vi "medicaoIXV.vi"() -> ()   [LabVIEW 2012]
uses:
  <vilib>/Utility/file.llb/Write To Spreadsheet File (string).vi
  <vilib>/Utility/file.llb/Write To Spreadsheet File (DBL).vi
  <instrlib>/Agilent 6XXX Series/Agilent 6XXX Series.lvlib
panel:
  out "reset graph":bool=TRUE
  out "tabela":dbl[][](array[numeric])
  in  "Tab Control":enum32{"Entrada de dados", "Saída de dados"}(tab)
  in  "nMedições":i16=1 caption="N° medições" min=1
  in  "area":dbl caption="Área da célula"
  in  "Tipo":string caption="Tipo da célula"
  in  "Formato":u16(ring) items=[".txt", ".csv"]
  out "ON/OFF1":bool caption="ON/OFF"
  in  "Pontos":dbl
  in  "Tensão máxima":dbl
  in  "Nome da célula":string
  in  "Local":path
  in  "Delay(ms)":dbl
  in  "Start":bool
  in  "temperatura":dbl caption="Temperatura da célula"
  in  "stopProgram":bool caption="Parar Programa"
  out "Imp":dbl
  out "Vmp":dbl
  out "Pmp":dbl
  out "Icc (A)":dbl
  out "Vca (V)":dbl
  in  "Print Screen":bool
  out "IXV":cluster{"Y":dbl[], "Y":dbl[]}[](graph)
  out "output voltage":dbl
  out "Tensao Atual (V)":dbl
  out "Corrente Atual\n(A)":dbl
  out "Ponto Atual":i32
  out "tabela":dbl[][](array[numeric]) caption="TABELA DE DADOS\nTensão(Fonte)      Pontos             Tensao           Corrente" format="%0.3f"
  in  "stop":bool caption="Parar Medição"
  out "ON/OFF2":bool caption="ON/OFF"
  in  "CorrenteGraph":dbl
  in  "error in (no error)":errorcluster
  out "error out":errorcluster
  in  "TensaoGraph":dbl
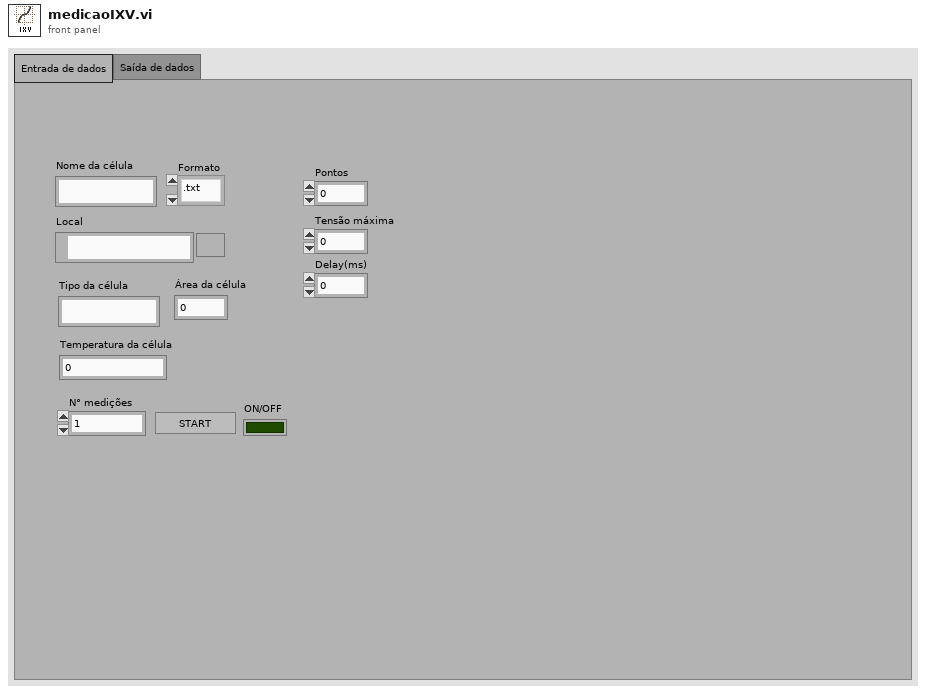
[diagram p1: front panel]
types:
  T1 = typedef "imagedata.ctl" = cluster{"image type":i32, "image depth":i32, "image":u8[], "mask":u8[], "colors":u32[], "Rectangle":cluster{"left":i16, "top":i16, "right":i16, "bottom":i16}}
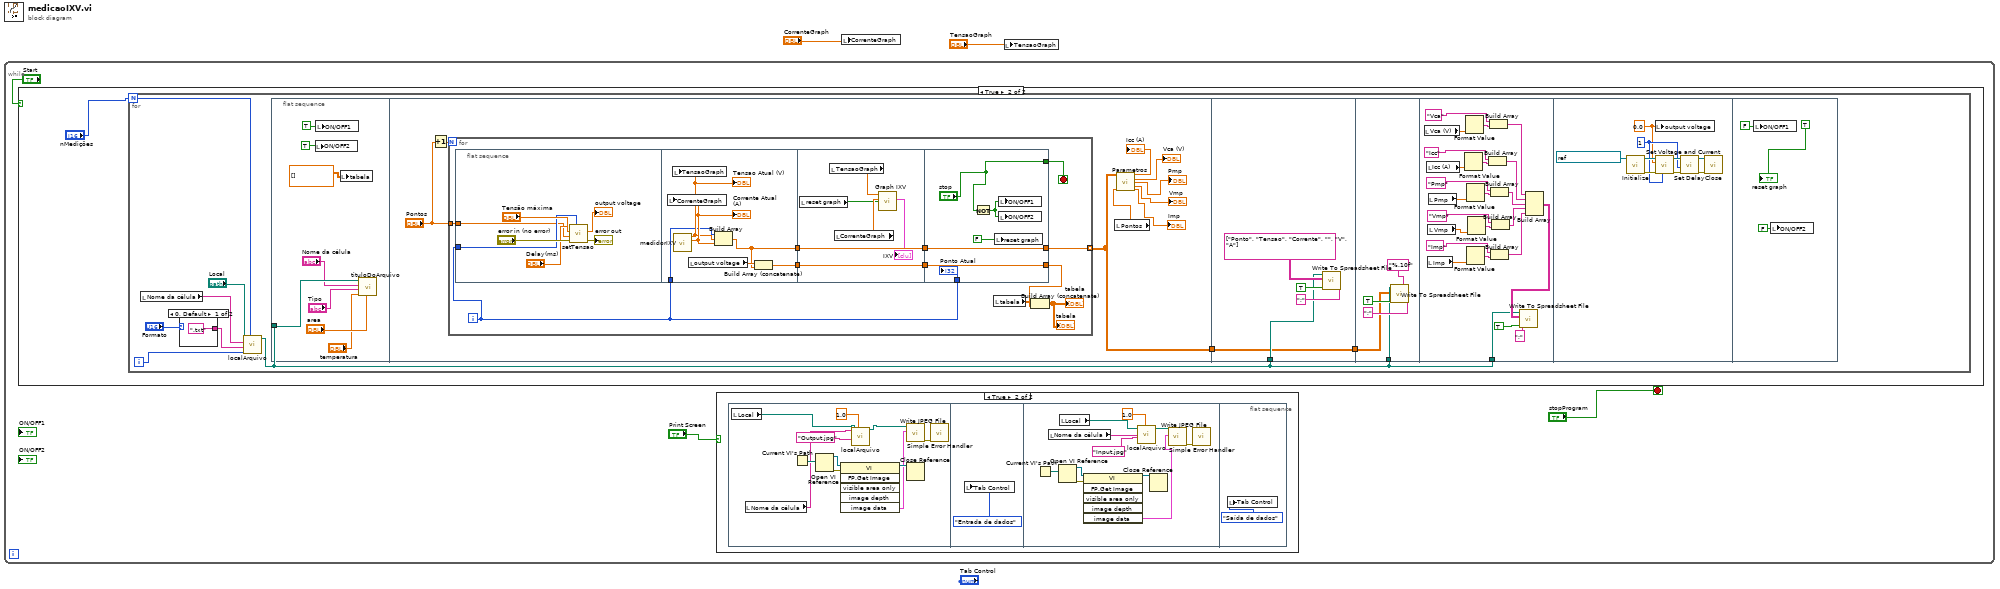
[diagram p0: block diagram]
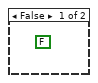
[diagram p3: hidden frame]
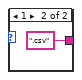
[diagram p4: hidden frame]
diagram:
  n1 = while {
    stop <- "stopProgram" stop-if-true
    n2 = case shown="True" "Start" {
      frame False {
        (unwired) FALSE
      }
      frame True {
        n3 = for {
          N: "nMedições" -> [w36]
          i -> [w32]
          n4 = local read "Nome da célula"() -> (w34:string)
          n5 = case shown="0, Default" "Formato" {
            tunnel: [".txt" ".csv"] -> w33
            frame 0, Default {
            }
            frame 1 {
            }
          }
          n6 = call "localArquivo.vi"("quantidadeDeArquivos"=w36, "numeroDoArquivo"=w32, "extensão"=w33, "Nome do arquivo"=w34, "Local"="Local") -> ("Path"=w31:path)  [unwired: 6 in]
          n7 = flat-sequence {
            tunnel: w31 -> [w49]
            tunnel: [w58] -> w39
            tunnel: w31 -> [w96]
            tunnel: [w95] -> w38
            tunnel: w39 -> [w95]
            tunnel: w31 -> [w101]
            tunnel: w38 -> [w100]
            tunnel: w31 -> [w105]
            frame #0 {
              n8 = local write "ON/OFF2"(TRUE ("ON/OFF2")) -> ()
              n9 = local write "ON/OFF1"(TRUE ("ON/OFF")) -> ()
              n10 = local write "tabela"(dbl[][] [] ("array")) -> ()
              n11 = call "tituloDoArquivo.vi"("area"="area", "temperatura"="temperatura", "Tipo"="Tipo", "Nome da célula"="Nome da célula", "file path (dialog if empty)"=w49) -> ()  [unwired: 7 in]
            }
            frame #1 {
              n12 = Increment(x="Pontos") -> (x+1=w57:dbl)
              n13 = for {
                N: w57 -> [_]
                tunnel: [w68] -> w58 mode=indexing
                tunnel: "Pontos" -> [w69]
                i -> [w62]
                stop <- w61 stop-if-true
                n14 = flat-sequence {
                  tunnel: w69 -> [w72]
                  tunnel: w62 -> [w73]
                  tunnel: w62 -> [w77]
                  tunnel: [w80] -> w67
                  tunnel: [w82] -> w66
                  tunnel: [w88] -> w60
                  tunnel: [w87] -> w59
                  tunnel: w66 -> [w87]
                  tunnel: w67 -> [w88]
                  tunnel: [w93] -> w65
                  tunnel: [w94] -> w68
                  tunnel: w60 -> [w94]
                  tunnel: w59 -> [w93]
                  tunnel: w62 -> [w92]
                  tunnel: ["stop"] -> w61
                  frame #0 {
                    n15 = call "setTensao.vi"("Ponto"=w73, "error in (no error)"="error in (no error)", "Pontos"=w72, "Tensão máxima"="Tensão máxima", "delay(ms)"="Delay(ms)") -> ("error out"=→"error out":errorcluster, "output voltage"=→"output voltage":dbl)  [unwired: 5 in]
                  }
                  frame #1 {
                    n16 = call "medidorIXV.vi"() -> ("Corrente Atual"=w79:dbl, "Tensao Atual"=w78:dbl)  [unwired: 10 in]
                    "Corrente Atual\n(A)" <- w79
                    "Tensao Atual (V)" <- w78
                    n17 = local write "CorrenteGraph"(w79) -> ()
                    n18 = local write "TensaoGraph"(w78) -> ()
                    n19 = local read "output voltage"() -> (w81:dbl)
                    n20 = Build Array(w77, w78, w79) -> (w80:dbl[])
                    n21 = Build Array (concatenate)(w81, w80) -> (w82:dbl[])
                  }
                  frame #2 {
                    n22 = local read "reset graph"() -> (w83:bool)
                    n23 = local read "TensaoGraph"() -> (w86:dbl)
                    n24 = local read "CorrenteGraph"() -> (w85:dbl)
                    n25 = call "Graph IXV"("Reset"=w83, "Y Input"=w85, "X Input"=w86) -> ("XY Graph"=→"IXV":cluster{"Y":dbl[], "Y":dbl[]}[])  [unwired: 2 in, 6 out]
                  }
                  frame #3 {
                    n26 = Not(x="stop") -> (.not. x?=w90:bool)
                    n27 = local write "reset graph"(FALSE) -> ()
                    n28 = local write "ON/OFF1"(w90) -> ()
                    n29 = local write "ON/OFF2"(w90) -> ()
                    "Ponto Atual" <- w92
                  }
                }
                n30 = local read "tabela"() -> (w64:dbl[][])
                n31 = Build Array (concatenate)(w64, w65) -> (→"tabela" →"tabela":dbl[][])
              }
              n32 = local read "Pontos"() -> (w55:dbl)
              n33 = call "Parametros.vi"("VetorDeDados"=w58, "pontos"=w55) -> ("Icc"=→"Icc (A)":dbl, "Vca"=→"Vca (V)":dbl, "Pmp"=→"Pmp":dbl, "Vmp"=→"Vmp":dbl, "Imp"=→"Imp":dbl)  [unwired: 9 in]
            }
            frame #2 {
              n34 = call-poly <vilib>:"Write To Spreadsheet File.vi"("delimiter (\\t)"=";" ("delimiter (\\t)"), "append to file? (new file:F)"=TRUE, "2D data"=string[][] [["Ponto", "Tensao", "Corrente"], ["", "V", "A"]], "file path (dialog if empty)"=w96) -> ()  [unwired: 4 in, 1 out]
            }
            frame #3 {
              n35 = call-poly <vilib>:"Write To Spreadsheet File.vi"("delimiter (\\t)"=";" ("delimiter (\\t)"), "format (%.3f)"="%.10f", "append to file? (new file:F)"=TRUE, "2D data"=w100, "file path (dialog if empty)"=w101) -> ()  [unwired: 3 in, 1 out]
            }
            frame #4 {
              n36 = local read "Vca (V)"() -> (w107:dbl)
              n37 = local read "Icc (A)"() -> (w117:dbl)
              n38 = local read "Imp"() -> (w120:dbl)
              n39 = local read "Vmp"() -> (w119:dbl)
              n40 = local read "Pmp"() -> (w118:dbl)
              n41 = Format Value(value (0)=w117) -> (output string=w110:string)  [unwired: 2 in]
              n42 = Format Value(value (0)=w107) -> (output string=w108:string)  [unwired: 2 in]
              n43 = Format Value(value (0)=w118) -> (output string=w112:string)  [unwired: 2 in]
              n44 = Format Value(value (0)=w120) -> (output string=w116:string)  [unwired: 2 in]
              n45 = Format Value(value (0)=w119) -> (output string=w114:string)  [unwired: 2 in]
              n46 = Build Array("Icc", w110) -> (w122:string[])
              n47 = Build Array("Vca", w108) -> (w121:string[])
              n48 = Build Array("Pmp", w112) -> (w123:string[])
              n49 = Build Array("Imp", w116) -> (w125:string[])
              n50 = Build Array("Vmp", w114) -> (w124:string[])
              n51 = Build Array(w121, w122, w123, w124, w125) -> (w126:string[][])
              n52 = call-poly <vilib>:"Write To Spreadsheet File.vi"("delimiter (\\t)"=";" ("delimiter (\\t)"), "append to file? (new file:F)"=TRUE, "2D data"=w126, "file path (dialog if empty)"=w105) -> ()  [unwired: 4 in, 1 out]
            }
            frame #5 {
              w129 = 0.0 ("voltage (0 V)")
              w132 = u8 1 ("channel (1)")
              n53 = call <instrlib>:"Initialize.vi"("VISA resource name"=refnum<visa-resource-name> "GPIB0::5::INSTR") -> ("error out"=w134:errorcluster, "VISA resource name out"=w133:refnum<visa-resource-name>)  [unwired: 9 in]
              n54 = local write "output voltage"(w129) -> ()
              n55 = call <instrlib>:"Set Voltage and Current.vi"("channel (1)"=w132, "error in (no error)"=w134, "voltage (0 V)"=w129, "VISA resource name"=w133) -> ("error out"=w135:errorcluster, "VISA resource name out"=w136:refnum<visa-resource-name>)  [unwired: 6 in]
              n56 = call <instrlib>:"Set Delay.vi"("error in (no error)"=w135, "channel (1)"=w132, "VISA resource name"=w136) -> ("error out"=w130:errorcluster, "VISA resource name out"=w131:refnum<visa-resource-name>)  [unwired: 7 in]
              n57 = call <instrlib>:"Close.vi"("error in (no error)"=w130, "VISA resource name"=w131) -> ()  [unwired: 9 in, 1 out]
            }
            frame #6 {
              n58 = local write "ON/OFF1"(FALSE) -> ()
              n59 = local write "ON/OFF2"(FALSE ("ON/OFF")) -> ()
              "reset graph" <- TRUE
            }
          }
        }
      }
    }
    n60 = case shown="True" "Print Screen" {
      frame False {
      }
      frame True {
        n61 = flat-sequence {
          frame #0 {
            n62 = local read "Local"() -> (w9:path)
            n63 = local read "Nome da célula"() -> (w7:string)
            n64 = Current VI's Path() -> (path=w14:path)
            n65 = Open VI Reference(vi path=w14) -> (vi reference=w15:refnum<vi>, error out=w16:errorcluster)  [unwired: 5 in]
            n66 = invoke class="VI" method="FP.Get Image"(reference=w15, error in=w16) -> (reference out=w13:refnum<vi>, "image data"=w12:T1)  [unwired: 4 in, 4 out]
            n67 = call "localArquivo.vi"("quantidadeDeArquivos"=1.0, "extensão"="Output.jpg", "Nome do arquivo"=w7, "Local"=w9) -> ("Path"=w6:path)  [unwired: 7 in]
            n68 = call <vilib>:"Write JPEG File.vi"("image data"=w12, "path to JPEG file"=w6) -> ("error out"=w11:errorcluster)  [unwired: 8 in, 1 out]
            n69 = Close Reference(reference=w13) -> ()  [unwired: 1 in, 1 out]
            n70 = call <vilib>:"Simple Error Handler.vi"("error in (no error)"=w11) -> ()  [unwired: 4 in, 5 out]
          }
          frame #1 {
            n71 = local write "Tab Control"(enum32{"Entrada de dados", "Saída de dados"}."Entrada de dados" ("Tab Control")) -> ()
          }
          frame #2 {
            n72 = Current VI's Path() -> (path=w27:path)
            n73 = local read "Nome da célula"() -> (w21:string)
            n74 = Open VI Reference(vi path=w27) -> (vi reference=w26:refnum<vi>, error out=w25:errorcluster)  [unwired: 5 in]
            n75 = local read "Local"() -> (w20:path)
            n76 = invoke class="VI" method="FP.Get Image"(reference=w26, error in=w25) -> (reference out=w28:refnum<vi>, "image data"=w23:T1)  [unwired: 4 in, 4 out]
            n77 = call "localArquivo.vi"("quantidadeDeArquivos"=1.0, "extensão"="Input.jpg", "Nome do arquivo"=w21, "Local"=w20) -> ("Path"=w19:path)  [unwired: 7 in]
            n78 = Close Reference(reference=w28) -> ()  [unwired: 1 in, 1 out]
            n79 = call <vilib>:"Write JPEG File.vi"("image data"=w23, "path to JPEG file"=w19) -> ("error out"=w24:errorcluster)  [unwired: 8 in, 1 out]
            n80 = call <vilib>:"Simple Error Handler.vi"("error in (no error)"=w24) -> ()  [unwired: 4 in, 5 out]
          }
          frame #3 {
            n81 = local write "Tab Control"(enum32{"Entrada de dados", "Saída de dados"}."Saída de dados" ("Tab Control")) -> ()
          }
        }
      }
    }
  }
  n82 = local write "CorrenteGraph"("CorrenteGraph") -> ()
  n83 = local write "TensaoGraph"("TensaoGraph") -> ()
